vi "Andor_Acquire.vi"(4 "AccDoneRef":refnum<vi>, 5 "IntegTime":u32=100 caption="Integration\nTime (ms)" min=1 max=100000 step=1, 6 "Stop Acq":refnum<vi>, 7 "Accumulation":u16=1 min=1 max=256 step=1, 8 "ErrorIn(NoErr)":errorcluster, 9 "Save":bool, 10 "AndorOpQ":refnum<queue>, 11 "AndorAcqQ":refnum<queue>) -> (0 "error out":errorcluster, 1 "Delta(ms)":u32, 2 "DeltaT":u32[](array[numeric]), 3 "Data out":i32[][](array[numeric]))   [LabVIEW 2019]
uses:
  Programmes Labview/LabScanV1A/DevicesClass/InstrumentsClass/AndorSpectro/AndorAcq_States.ctl
  <userlib>/atmcd32d.llb/Error Code Enum typedef.ctl
panel:
  in  "Stop Acq":bool
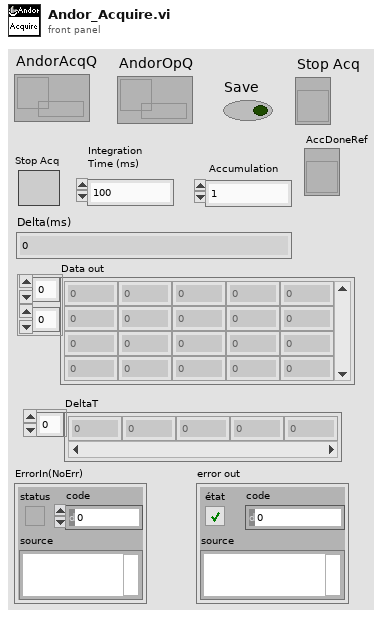
[diagram p1: front panel]
types:
  T1 = typedef "AndorAcq_States.ctl" = enum16{"Start", "Get Status", "Abort", "Error", "GetData"}
  T2 = typedef "Error Code Enum typedef.ctl" = enum32{"N/A (0)", "DRV_ERROR_CODES", "DRV_SUCCESS", "DRV_VXDNOTINSTALLED", "DRV_ERROR_SCAN", "DRV_ERROR_CHECK_SUM", "DRV_ERROR_FILELOAD", "DRV_UNKNOWN_FUNC", "DRV_ERROR_VXD_INIT", "DRV_ERROR_ADDRESS", "DRV_ERROR_PAGELOCK", "DRV_ERROR_PAGEUNLOCK", "DRV_ERROR_BOARDTEST", "DRV_ERROR_ACK", "DRV_ERROR_UP_FIFO", "DRV_ERROR_PATTERN", "N/A (16)", "DRV_ACQUISITION_ERRORS", "DRV_ACQ_BUFFER", "DRV_ACQ_DOWNFIFO_FULL", "DRV_PROC_UNKONWN_INSTRUCTION", "DRV_ILLEGAL_OP_CODE", "DRV_KINETIC_TIME_NOT_MET", "DRV_ACCUM_TIME_NOT_MET", "DRV_NO_NEW_DATA", "N/A (25)", "DRV_SPOOLERROR", "N/A (27)", "N/A (28)", "N/A (29)", "N/A (30)", "N/A (31)", "N/A (32)", "DRV_TEMPERATURE_CODES", "DRV_TEMPERATURE_OFF", "DRV_TEMPERATURE_NOT_STABILIZED", "DRV_TEMPERATURE_STABILIZED", "DRV_TEMPERATURE_NOT_REACHED", "DRV_TEMPERATURE_OUT_RANGE", "DRV_TEMPERATURE_NOT_SUPPORTED", "DRV_TEMPERATURE_DRIFT", "N/A (41)", "N/A (42)", "N/A (43)", "N/A (44)", "N/A (45)", "N/A (46)", "N/A (47)", "N/A (48)", "DRV_GENERAL_ERRORS", "DRV_INVALID_AUX", "DRV_COF_NOTLOADED", "DRV_FPGAPROG", "DRV_FLEXERROR", "DRV_GPIBERROR", "N/A (55)", "N/A (56)", "N/A (57)", "N/A (58)", "N/A (59)", "N/A (60)", "N/A (61)", "N/A (62)", "N/A (63)", "DRV_DATATYPE", "DRV_DRIVER_ERRORS", "DRV_P1INVALID", "DRV_P2INVALID", "DRV_P3INVALID", "DRV_P4INVALID", "DRV_INIERROR", "DRV_COFERROR", "DRV_ACQUIRING", "DRV_IDLE", "DRV_TEMPCYCLE", "DRV_NOT_INITIALIZED", "DRV_P5INVALID", "DRV_P6INVALID", "DRV_INVALID_MODE", "DRV_INVALID_FILTER", "DRV_I2CERRORS", "DRV_I2CDEVNOTFOUND", "DRV_I2CTIMEOUT", "DRV_P7INVALID", "N/A (84)", "N/A (85)", "N/A (86)", "N/A (87)", "N/A (88)", "N/A (89)", "DRV_IOCERROR", "DRV_VRMVERSIONERROR"}
  T3 = cluster{"Message":string, "Data":variant, "Code":i32}
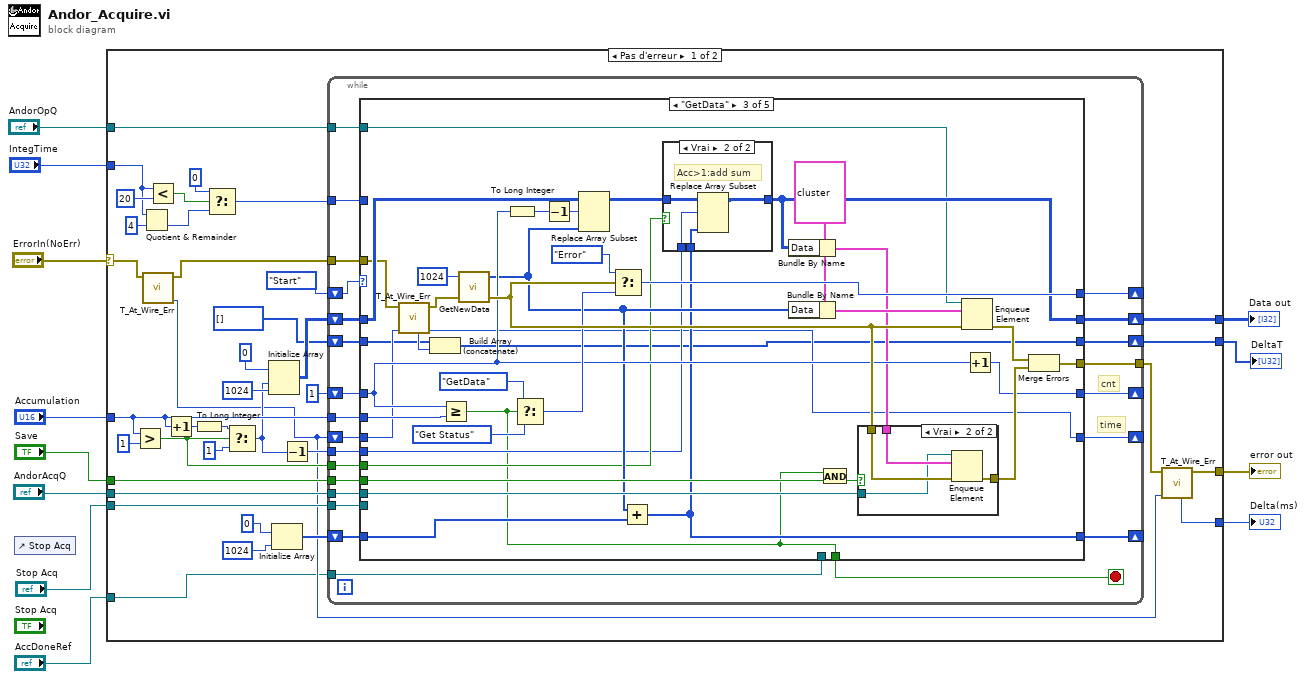
[diagram p0: block diagram]
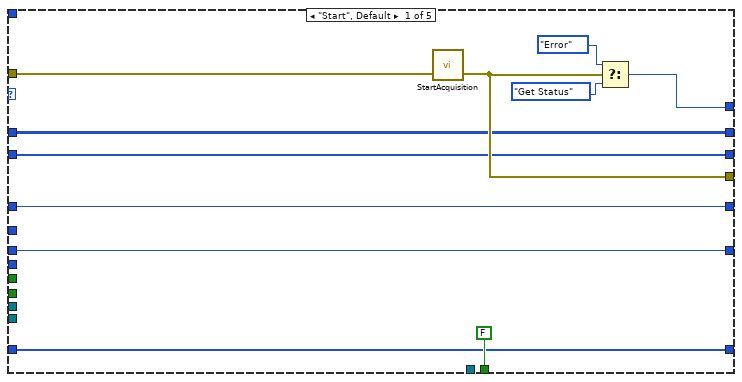
[diagram p2: hidden frame]
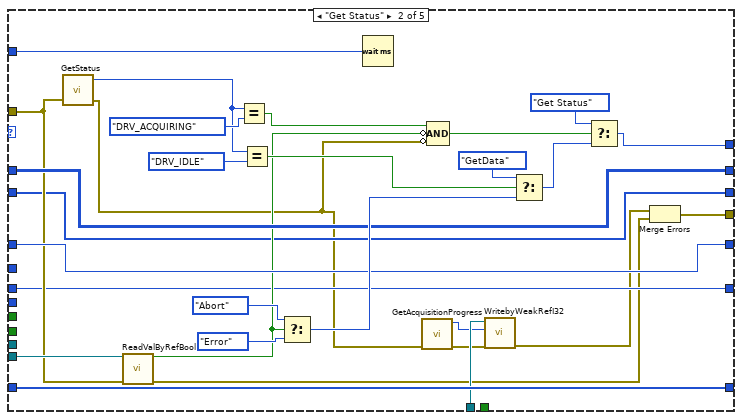
[diagram p3: hidden frame]
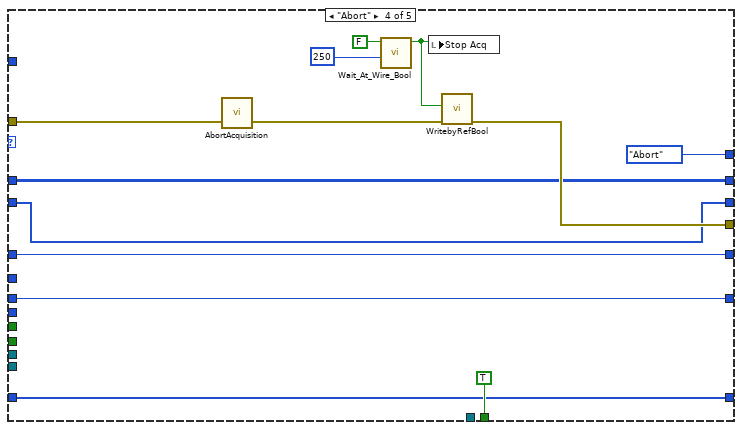
[diagram p6: hidden frame]
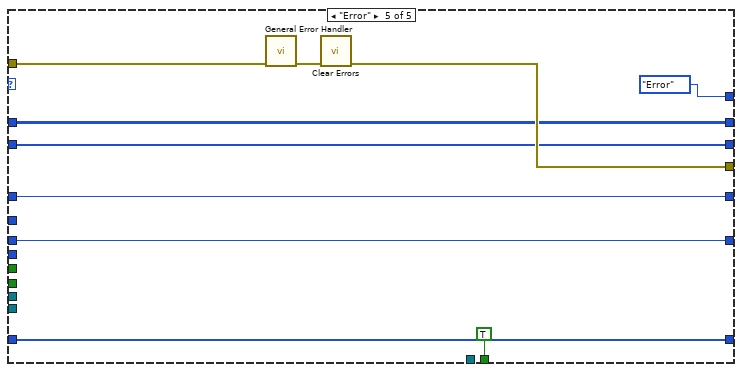
[diagram p7: hidden frame]
diagram:
  n1 = control-ref of="Stop Acq"() -> ()  [unwired: 1 out]
  n2 = case shown="Pas d'erreur" "ErrorIn(NoErr)" {
    selector: "ErrorIn(NoErr)" -> [w19 w185]
    tunnel: [w16 w185] -> w11
    tunnel: "AndorAcqQ" -> [w48 _]
    tunnel: "AndorOpQ" -> [w47 _]
    tunnel: "Save" -> [w46 _]
    tunnel: "Accumulation" -> [w33 _]
    tunnel: "Stop Acq" -> [w44 _]
    tunnel: "IntegTime" -> [w22 _]
    tunnel: [w36 _] -> w4
    tunnel: [w20 _] -> w3
    tunnel: [w14 _] -> w2
    tunnel: "AccDoneRef" -> [w13 _]
    frame No Error {
      n3 = Greater?(x=w33, y=u16 1) -> (0:w26:bool)
      n4 = Quotient & Remainder(x=w22, y=u32 4) -> (floor(x/y)=w42:u32)  [unwired: 1 out]
      n5 = call <userlib>:"T_At_Wire_Err.vi"("error in (no error)"=w19) -> ("Clock(ms)"=w15:u32, "error out"=w18:errorcluster)  [unwired: 8 in, 1 out]
      n6 = Less?(x=w22, y=u32 20 ("limite supérieure")) -> (x < y?=w23:bool)
      n7 = Increment(x=w33) -> (x+1=w32:u16)
      n8 = To Long Integer(number=w32) -> (32bit integer=w31:i32)
      n9 = Select(t=u32 0 ("cas vrai"), s=w23, f=w42) -> (s? t:f=w41:u32)
      n10 = Select(t=w31, s=w26, f=1 ("y")) -> (s? t:f=w27:i32)
      n11 = Initialize Array(0 ("élément"), w27, 1024 ("taille de la dimension")) -> (w37:i32[][])
      n12 = Initialize Array(0 ("élément"), 1024 ("taille de la dimension")) -> (w28:i32[])
      n13 = Decrement(x=w27) -> (x-1=w25:i32)
      n14 = while {
        tunnel: [w73] -> w17
        tunnel: w18 -> [w71]
        shift-right: [w70] -> _
        shift-left: AndorAcq_States."Start" ("AndorAcqSt") -> [w72]
        tunnel: w47 -> [w68]
        tunnel: w48 -> [w67]
        tunnel: w46 -> [w66]
        tunnel: w33 -> [w65]
        shift-right: [w63] -> _
        shift-left: u16 1 -> [w64]
        tunnel: w44 -> [w62]
        tunnel: w41 -> [w61]
        shift-right: [w59] -> w36
        shift-left: w37 -> [w60]
        shift-right: [w57] -> _
        shift-left: w28 -> [w58]
        tunnel: w25 -> [w56]
        tunnel: w26 -> [w55]
        shift-right: [w51] -> _
        shift-left: w15 -> [w54]
        shift-right: [w53] -> w20
        shift-left: u32[] [] -> [w52]
        tunnel: w13 -> [w50]
        stop <- w69 stop-if-true
        # "cnt"
        # "time"
        n15 = case shown="\"GetData\"" w72 {
          tunnel: [w82 w94 w145 w167 w180] -> w73
          tunnel: w71 -> [w76 w95 w123 w174 w184]
          tunnel: [w81 w111 w151 AndorAcq_States."Abort" ("AndorAcqSt") AndorAcq_States."Error" ("AndorAcqSt")] -> w70
          tunnel: [FALSE _ w114 TRUE TRUE] -> w69
          tunnel: w68 -> [_ _ w119 _ _]
          tunnel: w67 -> [_ _ w148 _ _]
          tunnel: w66 -> [_ _ w143 _ _]
          tunnel: w65 -> [_ _ w127 _ _]
          tunnel: w64 -> [w79 w104 w136 w166 w179]
          tunnel: [w79 w104 w138 w166 w179] -> w63
          tunnel: w62 -> [_ w97 _ _ _]
          tunnel: w61 -> [_ w99 _ _ _]
          tunnel: w60 -> [w78 w98 w137 w165 w178]
          tunnel: [w78 w98 w124 w165 w178] -> w59
          tunnel: w58 -> [w77 w93 w130 w164 w177]
          tunnel: [w77 w93 w128 w164 w177] -> w57
          tunnel: w56 -> [_ _ w125 _ _]
          tunnel: w55 -> [_ _ w126 _ _]
          tunnel: [w75 w92 w120 w163 w176] -> w51
          tunnel: w54 -> [w75 w92 w121 w163 w176]
          tunnel: [w74 w91 w117 w162 w175] -> w53
          tunnel: w52 -> [w74 w91 w116 w162 w175]
          tunnel: w50 -> [_ w90 _ _ _]
          frame "Start", Default {
            n16 = call <userlib>:"StartAcquisition.vi"("error in (no error)"=w76) -> ("error out"=w82:errorcluster)  [unwired: 1 in, 1 out]
            n17 = Select(t=AndorAcq_States."Error" ("AndorAcqSt"), s=w82, f=AndorAcq_States."Get Status" ("AndorAcqSt")) -> (s? t:f=w81:T1)
          }
          frame "Get Status" {
            n18 = call <userlib>:"GetStatus.vi"("error in (no error)"=w95) -> ("error out"=w87:errorcluster, "status"=w109:T2)  [unwired: 2 in, 1 out]
            n19 = call <userlib>:"ReadValByRefBool.vi"("Control Ref"=w97, "error in"=w95) -> ("Valeur"=w96:bool, "error out"=w85:errorcluster)  [unwired: 12 in]
            n20 = Equal?(x=w109, y=Error_Code_Enum_typedef."DRV_ACQUIRING" ("status")) -> (x = y?=w112:bool)
            n21 = Equal?(x=w109, y=Error_Code_Enum_typedef."DRV_IDLE" ("status")) -> (x = y?=w107:bool)
            n22 = Select(t=AndorAcq_States."Abort" ("AndorAcqSt"), s=w96, f=AndorAcq_States."Error" ("AndorAcqSt")) -> (s? t:f=w106:T1)
            n23 = Wait (ms)(milliseconds to wait=w99) -> ()  [unwired: 1 out]
            n24 = call <userlib>:"GetAcquisitionProgress.vi"("error in (no error)"=w87) -> ("error out"=w88:errorcluster, "accum"=w89:i32)  [unwired: 3 in, 2 out]
            n25 = Compound Arithmetic op=AND ("Opérateur arithmétique")(w112, invert w96, invert w87) -> (w110:bool)
            n26 = call <userlib>:"WritebyWeakRefI32.vi"("error in"=w88, "Valeur"=w89, "Control Ref"=w90) -> ("error out"=w86:errorcluster)  [unwired: 8 in]
            n27 = Select(t=AndorAcq_States."GetData" ("AndorAcqSt"), s=w107, f=w106) -> (s? t:f=w105:T1)
            n28 = Select(t=AndorAcq_States."Get Status" ("AndorAcqSt"), s=w110, f=w105) -> (s? t:f=w111:T1)
            n29 = Merge Errors(w86, w85) -> (w94:errorcluster)
          }
          frame "GetData" {
            w133 = T3 {"Message"="PlotSgl", "Data"=variant, "Code"=1}
            n30 = call <userlib>:"T_At_Wire_Err.vi"("InitClock(ms)"=w121, "error in (no error)"=w123) -> ("Clock(ms)"=w120:u32, "error out"=w122:errorcluster, "Delta(ms)"=w118:u32)  [unwired: 7 in]
            n31 = Build Array (concatenate)(w116, w118) -> (w117:u32[])
            n32 = Greater Or Equal?(x=w136, y=w127) -> (x >= y?=w114:bool)
            n33 = call <userlib>:"GetNewData.vi"("error in (no error)"=w122, "size"=u32 1024) -> ("error out"=w146:errorcluster, "array"=w131:i32[])  [unwired: 1 in, 1 out]
            n34 = To Long Integer(number=w136) -> (32bit integer=w134:i32)
            n35 = Select(t=AndorAcq_States."GetData" ("AndorAcqSt"), s=w114, f=AndorAcq_States."Get Status" ("AndorAcqSt")) -> (s? t:f=w139:T1)
            n36 = Decrement(x=w134) -> (x-1=w135:i32)
            n37 = Replace Array Subset(array=w137, new element=w131, index (row)=w135) -> (w129:i32[][])  [unwired: 1 in]
            n38 = Select(t=AndorAcq_States."Error" ("AndorAcqSt"), s=w146, f=w139) -> (s? t:f=w151:T1)
            n39 = Add(x=w131, y=w130) -> (x+y=w128:i32[])
            n40 = case shown="Vrai" w126 {
              tunnel: w129 -> [w152 w156]
              tunnel: w128 -> [_ w155]
              tunnel: w125 -> [_ w154]
              tunnel: [w152 w153] -> w124
              frame False {
              }
              frame True {
                # "Acc>1:add sum"
                n41 = Replace Array Subset(array=w156, new element=w155, index (row)=w154) -> (w153:i32[][])  [unwired: 1 in]
              }
            }
            n42 = Bundle By Name(cluster=w133, "Data"=w124) -> (w132:T3)
            n43 = Bundle By Name(cluster=w133, "Data"=w131) -> (w147:T3)
            n44 = And(x=w114, y=w143) -> (x .and. y?=w115:bool)
            n45 = case shown="Vrai" w115 {
              tunnel: w148 -> [_ w158]
              tunnel: w132 -> [_ w161]
              tunnel: w146 -> [w157 w160]
              tunnel: [w157 w159] -> w144
              frame False {
              }
              frame True {
                n46 = Enqueue Element(queue=w158, element=w161, error in (no error)=w160) -> (error out=w159:errorcluster)  [unwired: 1 in, 2 out]
              }
            }
            n47 = Enqueue Element(queue=w119, element=w147, error in (no error)=w146) -> (error out=w149:errorcluster)  [unwired: 1 in, 2 out]
            n48 = Increment(x=w136) -> (x+1=w138:u16)
            n49 = Merge Errors(w149, w144) -> (w145:errorcluster)
          }
          frame "Abort" {
            n50 = call <userlib>:"AbortAcquisition.vi"("error in (no error)"=w174) -> ("error out"=w169:errorcluster)  [unwired: 1 in, 1 out]
            n51 = call <userlib>:"Wait_At_Wire_Bool.vi"("Wait (ms)"=u32 250, "error in (no error)"=FALSE) -> ("error out"=w168:bool)  [unwired: 7 in, 2 out]
            n52 = local write "Stop Acq"(w168) -> ()
            n53 = call <userlib>:"WritebyRefBool.vi"("error in"=w169, "Valeur"=w168) -> ("error out"=w167:errorcluster)  [unwired: 9 in]
          }
          frame "Error" {
            n54 = call <vilib>:"General Error Handler.vi"("error in (no error)"=w184) -> ("error out"=w183:errorcluster)  [unwired: 10 in, 4 out]
            n55 = call <vilib>:"Clear Errors.vi"("error in (no error)"=w183) -> ("error out"=w180:errorcluster)  [unwired: 5 in, 1 out]
          }
        }
      }
      n56 = call <userlib>:"T_At_Wire_Err.vi"("InitClock(ms)"=w15, "error in (no error)"=w17) -> ("error out"=w16:errorcluster, "Delta(ms)"=w14:u32)  [unwired: 7 in, 1 out]
    }
    frame Error {
    }
  }
  "error out" <- w11
  "Data out" <- w4
  "DeltaT" <- w3
  "Delta(ms)" <- w2
